vi "未命名 1.vi"() -> ()   [LabVIEW 2012]
panel:
  in  "停止按钮":bool
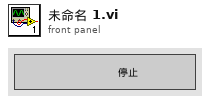
[diagram p1: front panel]
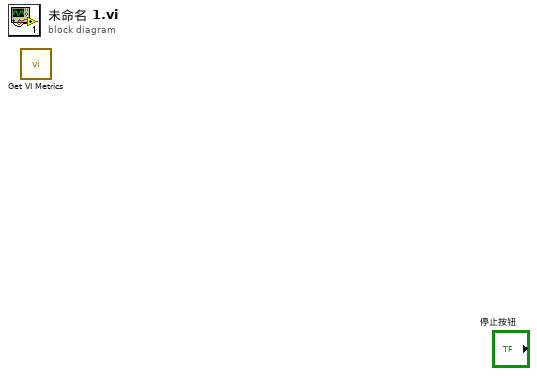
[diagram p0: block diagram]
diagram:
  n1 = call "Get VI Metrics.vi"() -> ()  [unwired: 12 in]
